vi "Explore_Open.vi"(7 "JPG":refnum<vi>, 8 "Task":enum16{"run", "open"}(ring), 10 "Name":string, 11 "String in":refnum<vi>) -> ()   [LabVIEW 2021]
panel:
  out "JPG":picture
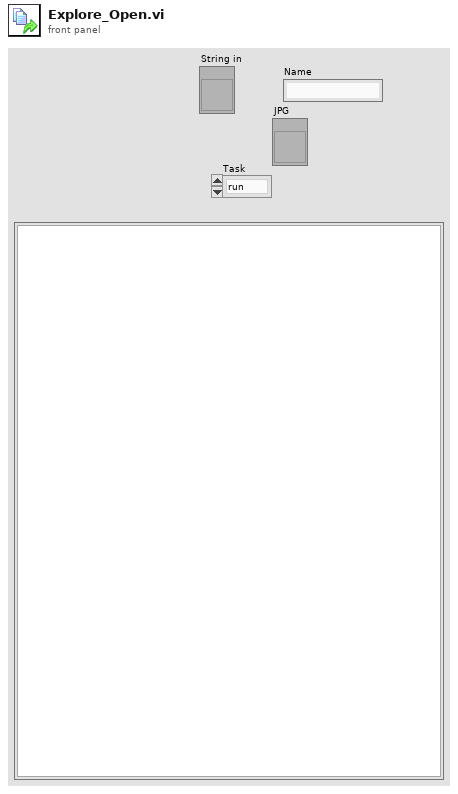
[diagram p1: front panel]
types:
  T1 = enum32{"Invalid", "Standard", "Closed", "Hidden", "Minimized", "Maximized"}
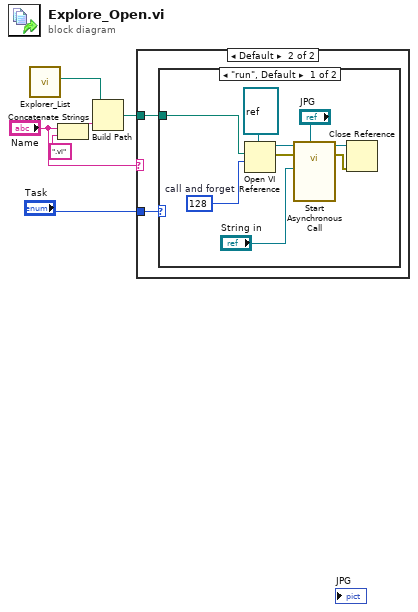
[diagram p0: block diagram]
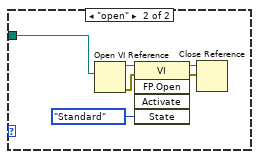
[diagram p3: hidden frame]
diagram:
  n1 = call "Explorer_List.vi"() -> ("Explore Path"=w6:path)  [unwired: 9 in, 2 out]
  n2 = Concatenate Strings("Name", ".vi" ("string")) -> (w2:string)
  n3 = Build Path(base path=w6, name or relative path=w2) -> (appended path=w5:path)
  n4 = case shown="Default" "Name" {
    tunnel: w5 -> [_ w8]
    tunnel: "Task" -> [_ w7]
    frame "" {
    }
    frame Default {
      n5 = case shown="\"run\", Default" w7 {
        tunnel: w8 -> [w10 w23]
        frame "run", Default {
          w16 = 128  # call and forget
          n6 = Open VI Reference(type specifier VI Refnum (for type only)=refnum<vi> refnum, vi path=w10, options=w16) -> (vi reference=w11:refnum<vi>, error out=w14:errorcluster)  [unwired: 3 in]
          n7 = call-by-ref "Start Asynchronous Call"(reference=w11, error in=w14, "JPG"="JPG", "Console Reference"="String in") -> (reference out=w13:refnum<vi>, error out=w12:errorcluster)  [unwired: 10 in]
          n8 = Close Reference(reference=w13, error in (no error)=w12) -> ()  [unwired: 1 out]
        }
        frame "open" {
          n9 = Open VI Reference(vi path=w23) -> (vi reference=w22:refnum<vi>, error out=w21:errorcluster)  [unwired: 5 in]
          n10 = invoke class="VI" method="FP.Open"(reference=w22, error in=w21, "State"=T1."Standard") -> (reference out=w20:refnum<vi>, error out=w19:errorcluster)  [unwired: 2 in, 3 out]
          n11 = Close Reference(reference=w20, error in (no error)=w19) -> ()  [unwired: 1 out]
        }
      }
    }
  }
